vi "main.vi"() -> ()   [LabVIEW 2023]
panel:
  out "error out 2":errorcluster
  in  "stop":bool
  out "error out":errorcluster
  in  "?":refnum<visa-resource-name>
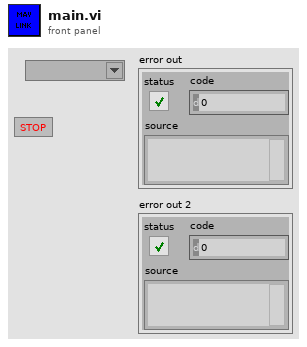
[diagram p1: front panel]
types:
  T1 = cluster{"len":u8, "incompat_flags":u8, "compat_flags":u8, "seq":u8, "sysid":u8, "compid":u8, "msgid":u32, "magic":u8, "payload":string, "checksum":u16, "signature":string}
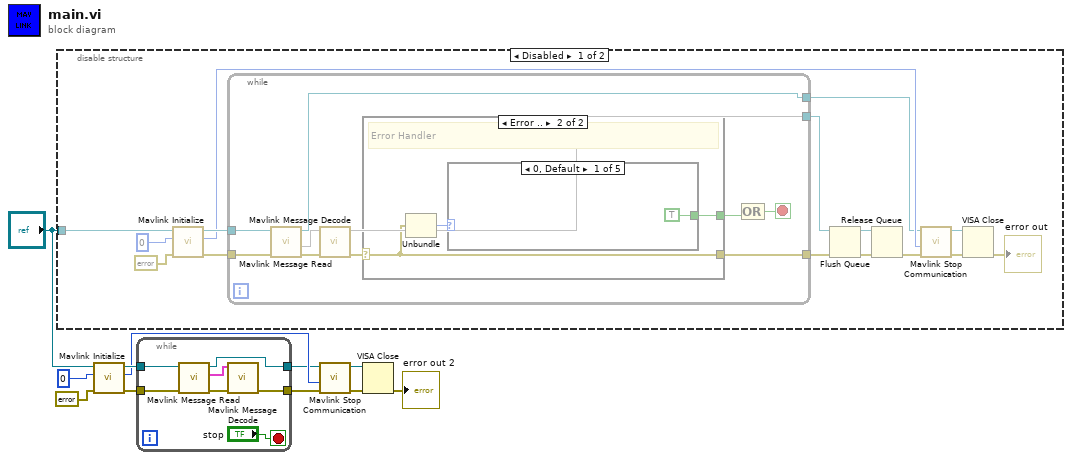
[diagram p0: block diagram]
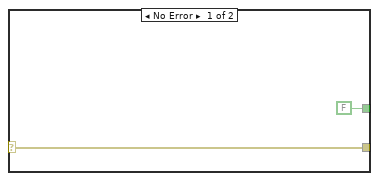
[diagram p2: hidden frame]
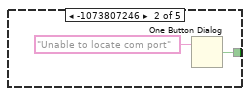
[diagram p3: hidden frame]
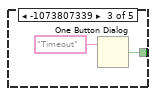
[diagram p4: hidden frame]
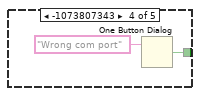
[diagram p5: hidden frame]
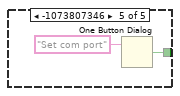
[diagram p6: hidden frame]
diagram:
  n1 = disable-structure shown="Disabled" {
    disable-tunnel: "?" -> [w12 _]
    frame Disabled {
      n2 = call "Mavlink Initialize.vi"("error in"=errorcluster {"status"=FALSE, "code"=0, "source"=""}, "Packet Sequence In"=u8 0, "VISA in"=w12) -> ("Error Out"=w25:errorcluster, "Packet Sequence Out"=w24:u8, "VISA resource name Out"=w26:refnum<visa-resource-name>)  [unwired: 5 in]
      n3 = while {
        tunnel: [w35] -> w23
        tunnel: w26 -> [w37]
        tunnel: [w33] -> w21
        tunnel: w25 -> [w36]
        tunnel: [w34] -> w22
        stop <- w28 stop-if-true
        n4 = call "Mavlink Message Read.vi"("error_in"=w36, "VISA In"=w37) -> ("error_out"=w32:errorcluster, 1:w27, "VISA Out"=w33:refnum<visa-resource-name>)  [unwired: 6 in, 1 out]
        n5 = call "Mavlink Message Decode.vi"("mav_msg"=w27, "error_in"=w32) -> (7:w35, "error_out"=w31:errorcluster)  [unwired: 7 in]
        n6 = case shown="Error .." w31 {
          selector: w31 -> [w38 w41]
          tunnel: [FALSE ("y") w40] -> w29
          tunnel: [w38 w41] -> w34
          frame No Error {
          }
          frame Error {
            # "Error Handler"
            n7 = Unbundle(w41) -> ("code"=w42:i32)  [unwired: 2 out]
            n8 = case shown="0, Default" w42 {
              tunnel: [TRUE ("true") w45 w47 w49 w51] -> w40
              frame 0, Default {
              }
              frame -1073807246 {
                n9 = One Button Dialog(message="Unable to locate com port") -> (true=w45:bool)  [unwired: 1 in]
              }
              frame -1073807339 {
                n10 = One Button Dialog(message="Timeout") -> (true=w47:bool)  [unwired: 1 in]
              }
              frame -1073807343 {
                n11 = One Button Dialog(message="Wrong com port") -> (true=w49:bool)  [unwired: 1 in]
              }
              frame -1073807346 {
                n12 = One Button Dialog(message="Set com port") -> (true=w51:bool)  [unwired: 1 in]
              }
            }
          }
        }
        n13 = Compound Arithmetic op=OR(w29) -> (w28:bool, w30:bool)
      }
      n14 = Flush Queue(queue=w23, error in (no error)=w22) -> (queue out=w16:refnum<queue>, error out=w15:errorcluster)  [unwired: 1 out]
      n15 = Release Queue(queue=w16, error in (no error)=w15) -> (error out=w17:errorcluster)  [unwired: 1 in, 2 out]
      n16 = call "Mavlink Stop Communication.vi"("error in (no error)"=w17, "Packet Sequence In"=w24, "VISA resource name"=w21) -> ("error out"=w19:errorcluster, "VISA resource name out"=w18:refnum<visa-resource-name>)  [unwired: 6 in, 1 out]
      n17 = VISA Close(VISA resource name=w18, error in (no error)=w19) -> (error out=→"error out":errorcluster)
    }
    frame Enabled {
    }
  }
  n18 = call "Mavlink Initialize.vi"("error in"=errorcluster {"status"=FALSE, "code"=0, "source"=""}, "Packet Sequence In"=u8 0, "VISA in"="?") -> ("Error Out"=w7:errorcluster, "Packet Sequence Out"=w4:u8, "VISA resource name Out"=w8:refnum<visa-resource-name>)  [unwired: 5 in]
  n19 = while {
    tunnel: w8 -> [w58]
    tunnel: [w56] -> w3
    tunnel: w7 -> [w57]
    tunnel: [w54] -> w2
    stop <- "stop" stop-if-true
    n20 = call "Mavlink Message Read.vi"("error_in"=w57, "VISA In"=w58) -> ("error_out"=w53:errorcluster, "mav_msg"=w52:T1, "VISA Out"=w56:refnum<visa-resource-name>)  [unwired: 7 in]
    n21 = call "Mavlink Message Decode.vi"("mav_msg"=w52, "error_in"=w53) -> ("error_out"=w54:errorcluster)  [unwired: 8 in]
  }
  n22 = call "Mavlink Stop Communication.vi"("error in (no error)"=w2, "Packet Sequence In"=w4, "VISA resource name"=w3) -> ("error out"=w6:errorcluster, "VISA resource name out"=w5:refnum<visa-resource-name>)  [unwired: 6 in, 1 out]
  n23 = VISA Close(VISA resource name=w5, error in (no error)=w6) -> (error out=→"error out 2":errorcluster)
